vi "Subvi AO trigger.vi"(8 "Trigger":bool, 10 "Enable trigger":bool) -> (2 "Scan direction":bool)   [LabVIEW 2017]
uses:
  <vilib>/Platform/TimedLoop/XDataNode/timing_clust.ctl
  <vilib>/Platform/TimedLoop/XDataNode/nitl_modes.ctl
  <vilib>/Platform/TimedLoop/XDataNode/wakeup.ctl
  <vilib>/rvi/Emulation/niFpgaSctlEmulationGetInTimedLoop.vi
  <vilib>/rvi/Emulation/niFpgaEmulationReportErrorSimple.vi
  <vilib>/rvi/Emulation/niFpgaGetClockAttributes.vi
  <vilib>/rvi/Emulation/niFpgaCriticalErrorInLSC.vi
  GV trigger delay.vi
  GV frame counter.vi
  <vilib>/Platform/TimedLoop/XDataNode/XDataNode.xnode
  <vilib>/Platform/TimedLoop/XDataNode/XDNodeRunTimeDep.lvlib
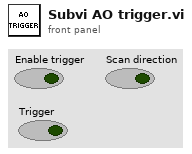
[diagram p1: front panel]
types:
  T1 = typedef "XDNodeRunTimeDep.lvlib/timing_clust.ctl" = cluster{"Expected End [f-1]":u64, "Actual End [f-1]":u64, "Finished Late? [f-1]":bool, "Expected End [i-1]":u64, "Actual End [i-1]":u64, "Finished Late? [i-1]":bool, "Expected Start [i]":u64, "Actual Start [i]":u64, "Expected Start [f]":u64, "Actual Start [f]":u64, "Source Name":string, "Structure Name":string, "Period":i64, "Deadline":i64, "Offset":i64, "Start":i64, "Priority":i32, "Timeout":i32, "Mode":T2, "Wakeup Reason":T3, "Error":errorcluster, "Source Type":string, "Secondary Source Type":string, "Global End Time":u64, "Global Start Time":u64, "Frame Duration":u64, "Iteration Duration":u64, "Assigned CPU":i32, "I/O Scan Engine Mode":u32}
  T2 = typedef "XDNodeRunTimeDep.lvlib/nitl_modes.ctl" = enum32{"No Change", "Process missed periods, maintain original phase", "Discard missed periods, maintain original phase", "Process missed periods, ignore original phase", "Discard missed periods, ignore original phase"}
  T3 = typedef "XDNodeRunTimeDep.lvlib/wakeup.ctl" = enum32{"Normal", "Aborted", "Asynchronous wakeup", "Timing source error", "Timed loop error", "Timeout"}
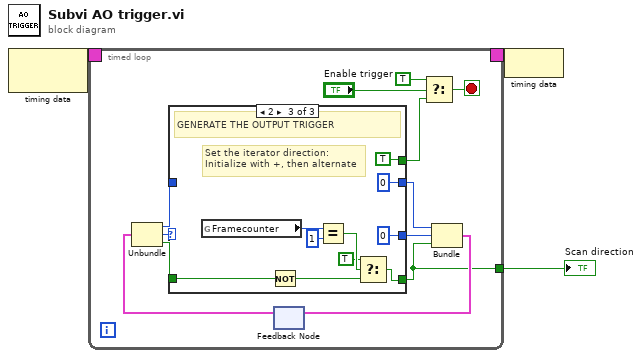
[diagram p0: block diagram]
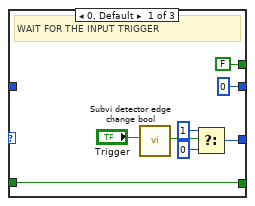
[diagram p2: hidden frame]
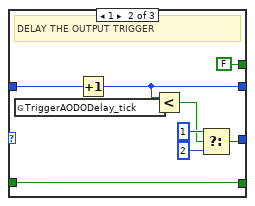
[diagram p3: hidden frame]
diagram:
  n1 = node-c288() -> (w3:T1)  [unwired: 1 in]
  n2 = timed-loop {
    timing: w3 -> [_]
    timing-out: [_] -> w2
    tunnel: [w4] -> w1
    stop <- w15 stop-if-true
    n3 = feedback #1() -> (w9:cluster{u16, "f":u8, bool})  [unwired: 1 in]
    n4 = Unbundle(w9) -> (w8:u16, "f"=w6:u8, w5:bool)
    n5 = case shown="2" w6 {
      tunnel: [u16 0 w30 u16 0] -> w12
      tunnel: [w23 w26 u8 0 ("f")] -> w7
      tunnel: w8 -> [_ w31 _]
      tunnel: [FALSE FALSE TRUE] -> w11
      tunnel: [w18 w24 w33] -> w4
      tunnel: w5 -> [w18 w24 w35]
      frame 0, Default {
        # "WAIT FOR THE INPUT TRIGGER"
        n6 = call "Subvi detector edge change bool.vi"("Input"="Trigger") -> ("Output"=w17:bool)  [unwired: 8 in]
        n7 = Select(t=u8 1, s=w17, f=u8 0) -> (s? t:f=w23:u8)
      }
      frame 1 {
        # "DELAY THE OUTPUT TRIGGER"
        n8 = global read "GV trigger delay.vi" "TriggerAODODelay_tick"() -> (w32:u16)
        n9 = Increment(x=w31) -> (x+1=w30:u16)
        n10 = Less?(x=w30, y=w32) -> (x < y?=w28:bool)
        n11 = Select(t=u8 1, s=w28, f=u8 2) -> (s? t:f=w26:u8)
      }
      frame 2 {
        # "Set the iterator direction:\nInitialize with +, then alternate"
        # "GENERATE THE OUTPUT TRIGGER"
        n12 = global read "GV frame counter.vi" "Framecounter"() -> (w37:u8)
        n13 = Not(x=w35) -> (.not. x?=w34:bool)
        n14 = Equal?(x=w37, y=u8 1) -> (x = y?=w39:bool)
        n15 = Select(t=TRUE, s=w39, f=w34) -> (s? t:f=w33:bool)
      }
    }
    n16 = Select(t=TRUE, s="Enable trigger", f=w11) -> (s? t:f=w15:bool)
    n17 = Bundle(w12, "f"=w7, w4) -> (w10:cluster{u16, "f":u8, bool})  [unwired: 1 in]
    n18 = feedback-in #1(w10) -> ()
  }
  "Scan direction" <- w1
  n19 = node-c288(w2) -> ()
